vi "oa_Process Block Size and Trigger Period.vi"(7 "dr":dbl=1.0, 8 "block size":i32=1024, 11 "trigger period [rev]":dbl=1.0) -> (0 "block size out":i32, 3 "trigger period out [rev]":dbl=1.0)   [LabVIEW 2017, in "SoundVib_OAUtility.lvlib"]
uses:
  <vilib>/addons/Sound and Vibration/Order Analysis/Utility/SoundVib_OAUtility.lvlib
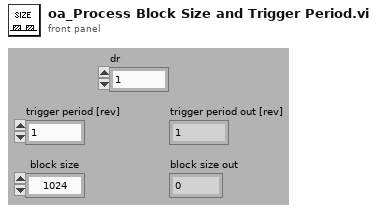
[diagram p1: front panel]
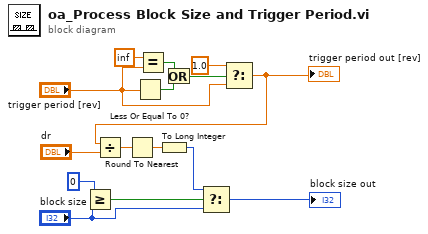
[diagram p0: block diagram]
diagram:
  n1 = Greater Or Equal?(x=0 ("y"), y="block size") -> (x >= y?=w15:bool)
  n2 = Less Or Equal To 0?(x="trigger period [rev]") -> (x <= 0?=w3:bool)
  n3 = Equal?(x=inf, y="trigger period [rev]") -> (x = y?=w4:bool)
  n4 = Or(x=w4, y=w3) -> (x .or. y?=w2:bool)
  n5 = Select(t=1.0, s=w2, f="trigger period [rev]") -> (s? t:f=w8:dbl)
  "trigger period out [rev]" <- w8
  n6 = Divide(x=w8, y="dr") -> (x/y=w13:dbl)
  n7 = Round To Nearest(number=w13) -> (nearest integer value=w12:dbl)
  n8 = To Long Integer(number=w12) -> (32bit integer=w11:i32)
  n9 = Select(t=w11, s=w15, f="block size") -> (s? t:f=→"block size out":i32)
